vi "LABVIEW TEST.vi"() -> ()   [LabVIEW 2019]
uses:
  <vilib>/Instr/_visa.llb/VISA Configure Serial Port (Instr).vi
panel:
  out "read buffer":string
  in  "baud rate (9600)":u32=9600
  out "String":string
  in  "stop":bool
  in  "LF":bool
  in  "LO":bool
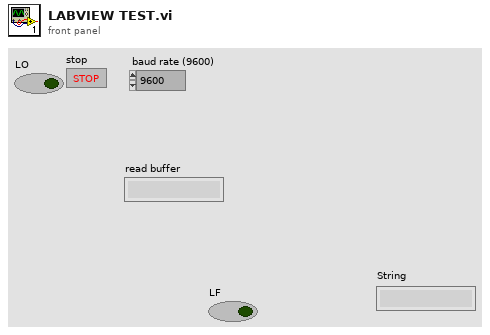
[diagram p1: front panel]
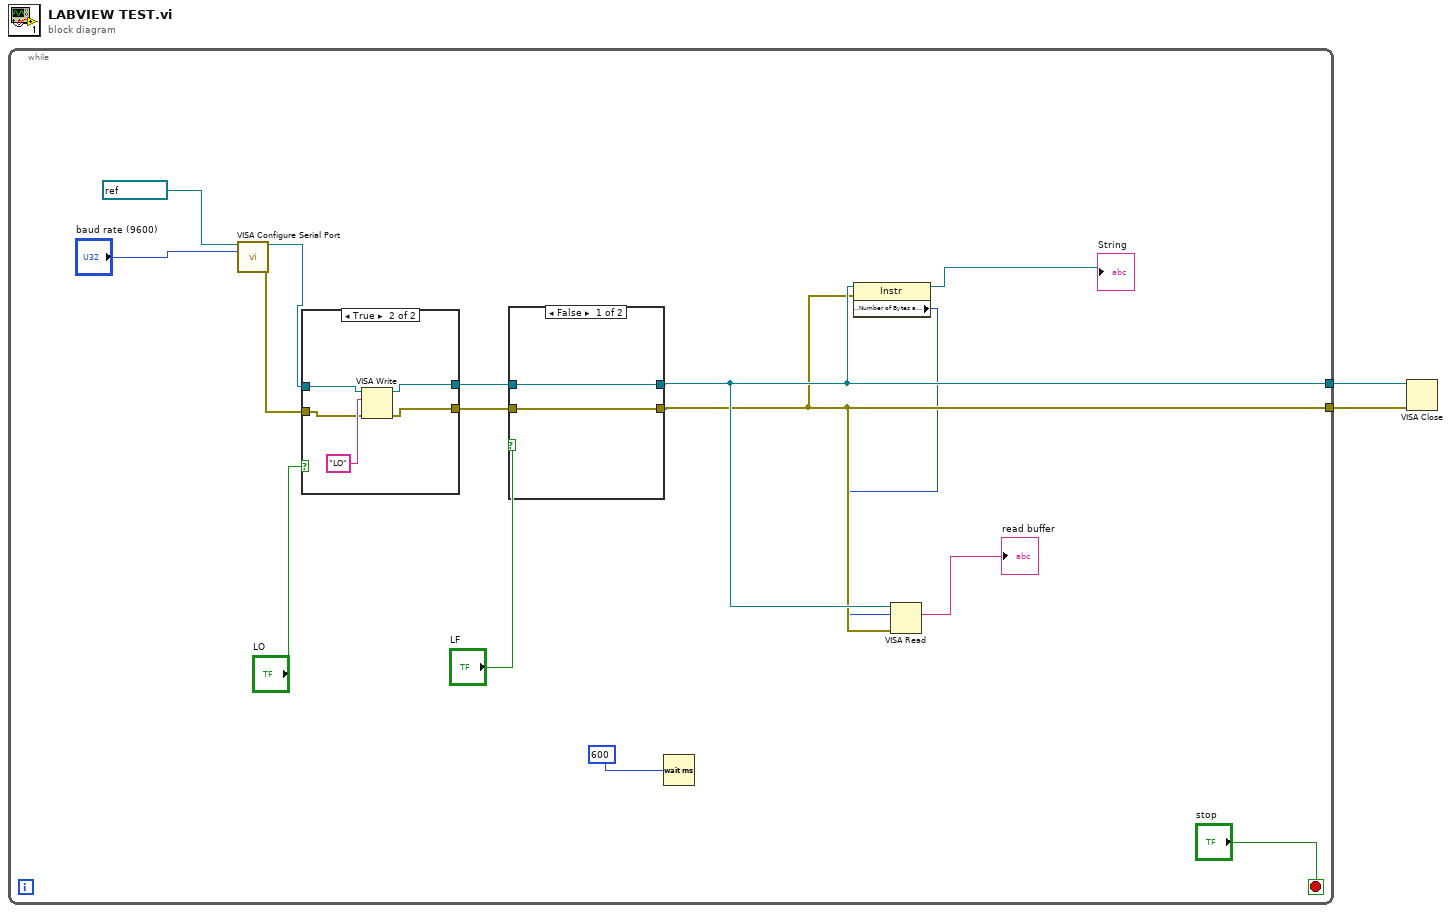
[diagram p0: block diagram]
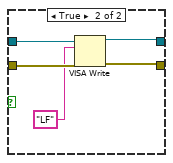
[diagram p2: hidden frame]
diagram:
  n1 = while {
    tunnel: [w6] -> w2
    tunnel: [w5] -> w1
    stop <- "stop" stop-if-true
    n2 = call-poly "VISA Configure Serial Port"("VISA resource name"=refnum<visa-resource-name> "COM6", "baud rate (9600)"="baud rate (9600)") -> ("VISA resource name out"=w12:refnum<visa-resource-name>, "error out"=w11:errorcluster)  [unwired: 12 in]
    n3 = case shown="True" "LO" {
      tunnel: w12 -> [w26 w31]
      tunnel: w11 -> [w25 w29]
      tunnel: [w26 w28] -> w17
      tunnel: [w25 w27] -> w16
      frame False {
      }
      frame True {
        n4 = VISA Write(VISA resource name=w31, write buffer="LO", error in (no error)=w29) -> (VISA resource name out=w28:refnum<visa-resource-name>, error out=w27:errorcluster)  [unwired: 1 out]
      }
    }
    n5 = case shown="False" "LF" {
      tunnel: w17 -> [w19 w24]
      tunnel: w16 -> [w18 w22]
      tunnel: [w19 w23] -> w6
      tunnel: [w18 w21] -> w5
      frame False {
      }
      frame True {
        n6 = VISA Write(VISA resource name=w24, write buffer="LF", error in (no error)=w22) -> (VISA resource name out=w23:refnum<visa-resource-name>, error out=w21:errorcluster)  [unwired: 1 out]
      }
    }
    n7 = Wait (ms)(milliseconds to wait=u32 600) -> ()  [unwired: 1 out]
    n8 = property class="Instr"(reference=w6, error in=w5) -> (reference out=→"String":refnum<visa-resource-name>, "Serial Settings:Number of Bytes at Serial Port"=w3:u32)  [unwired: 1 out]
    n9 = VISA Read(VISA resource name=w6, byte count=w3, error in (no error)=w5) -> (read buffer=→"read buffer":string)  [unwired: 3 out]
  }
  n10 = VISA Close(VISA resource name=w2, error in (no error)=w1) -> ()  [unwired: 1 out]
